vi "Car Main.vi"() -> ()   [LabVIEW 2014]
uses:
  <vilib>/Platform/TimedLoop/XDataNode/timing_clust.ctl
  <vilib>/Platform/TimedLoop/XDataNode/nitl_modes.ctl
  <vilib>/Platform/TimedLoop/XDataNode/wakeup.ctl
  <vilib>/FPGAPlugInAG/sbRIO-9626/niLvFpga_Open_sbRIO-9626.vi
  <vilib>/FPGAPlugInAG/sbRIO-9626/niLvFpga_Reset_sbRIO-9626.vi
  Global Data.vi
  <vilib>/Utility/error.llb/Error Cluster From Error Code.vi
  <vilib>/rvi/errors/niLvFpgaAdjustHostInterfaceError.vi
  <vilib>/FPGAPlugInAG/sbRIO-9626/niLvFpga_Close_sbRIO-9626.vi
  <vilib>/rvi/interface/nirviOpenFPGA/nirviOpenFPGA.xnode
  FPGA Bitfiles/FormulaElectric2_FPGATarget_FPGA_8a5J0mMac2U.lvbitx
  <vilib>/rvi/interface/nirviMethod/nirviMethod.xnode
  <vilib>/Platform/TimedLoop/XDataNode/XDataNode.xnode
  <vilib>/rvi/interface/nirviReadWriteControl/nirviReadWriteControl.xnode
  <vilib>/rvi/interface/nirviCloseFPGA/nirviCloseFPGA.xnode
  <vilib>/NI_Real-Time Target Support.lvlib
  <vilib>/Platform/TimedLoop/XDataNode/XDNodeRunTimeDep.lvlib
  NiFpgaLv.dll
panel:
  in  "baud rate (125000 bps)":u32=250000
  in  "Shutdown":bool
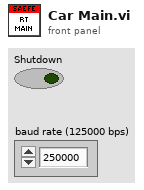
[diagram p1: front panel]
types:
  T1 = typedef "XDNodeRunTimeDep.lvlib/timing_clust.ctl" = cluster{"Expected End [f-1]":u64, "Actual End [f-1]":u64, "Finished Late? [f-1]":bool, "Expected End [i-1]":u64, "Actual End [i-1]":u64, "Finished Late? [i-1]":bool, "Expected Start [i]":u64, "Actual Start [i]":u64, "Expected Start [f]":u64, "Actual Start [f]":u64, "Source Name":string, "Structure Name":string, "Period":i64, "Deadline":i64, "Offset":i64, "Start":i64, "Priority":i32, "Timeout":i32, "Mode":T2, "Wakeup Reason":T3, "Error":errorcluster, "Source Type":string, "Secondary Source Type":string, "Global End Time":u64, "Global Start Time":u64, "Frame Duration":u64, "Iteration Duration":u64, "Assigned CPU":i32, "I/O Scan Engine Mode":u32}
  T2 = typedef "XDNodeRunTimeDep.lvlib/nitl_modes.ctl" = enum32{"No Change", "Process missed periods, maintain original phase", "Discard missed periods, maintain original phase", "Process missed periods, ignore original phase", "Discard missed periods, ignore original phase"}
  T3 = typedef "XDNodeRunTimeDep.lvlib/wakeup.ctl" = enum32{"Normal", "Aborted", "Asynchronous wakeup", "Timing source error", "Timed loop error", "Timeout"}
  T4 = typedef "Remote Stop Type.ctl" = cluster{"bRemoteStop":bool, "bRemoteEmergencyStop":bool, "bRemoteReturnToPits":bool, "bRemoteNewLogs":bool}
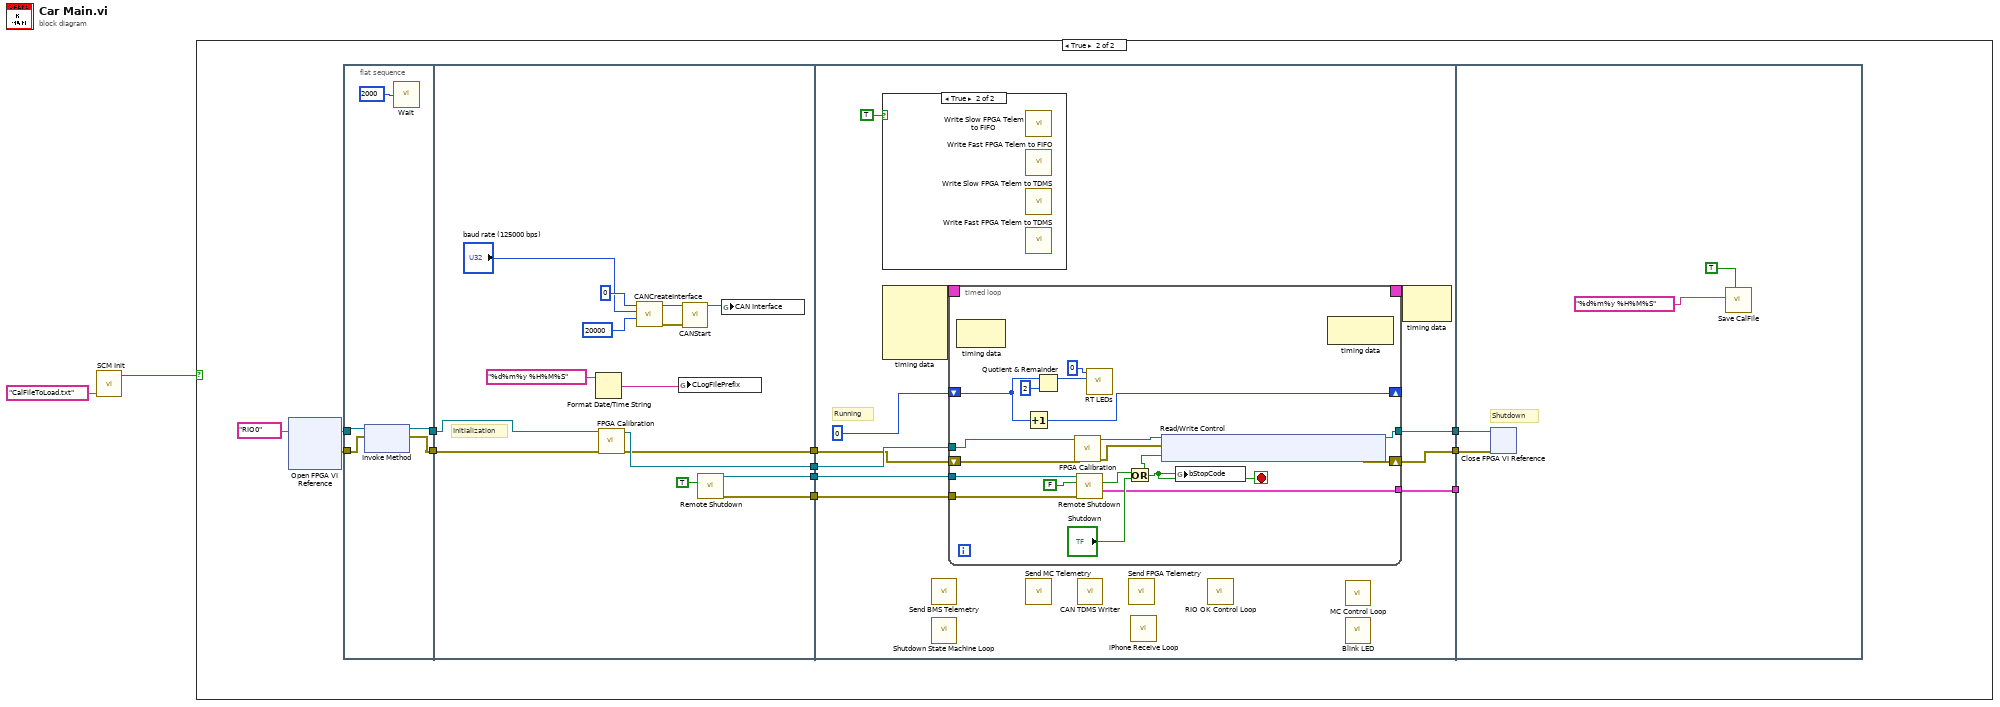
[diagram p0: block diagram]
diagram:
  n1 = call "SCM Init"("Calibration File"="CalFileToLoad.txt") -> ("InitOK"=w2:bool)  [unwired: 2 in, 2 out]
  n2 = case shown="True" w2 {
    frame False {
    }
    frame True {
      n3 = xnode "Open FPGA VI Reference"("resource name"=tag "RIO0") -> ("FPGA VI Reference Out"=w5:refnum<k20>, "error out"=w4:errorcluster)  [unwired: 1 in]
      n4 = flat-sequence {
        tunnel: w4 -> [w17]
        tunnel: w5 -> [w18]
        tunnel: [w16] -> w14
        tunnel: [w15] -> w13
        tunnel: [w21] -> w12
        tunnel: [w20] -> w11
        tunnel: [w33] -> w10
        tunnel: [w32] -> w9
        tunnel: w14 -> [w23]
        tunnel: w13 -> [w22]
        tunnel: w12 -> [w45]
        tunnel: w11 -> [w44]
        tunnel: w10 -> [w42]
        tunnel: w9 -> [w41]
        tunnel: [w40] -> w8
        tunnel: [w37] -> w7
        tunnel: [w36] -> w6
        tunnel: w8 -> [_]
        tunnel: w7 -> [w71]
        tunnel: w6 -> [w70]
        frame #0 {
          n5 = xnode "Invoke Method"("FPGA VI Reference In"=w18, "error in"=w17) -> ("FPGA VI Reference Out"=w16:refnum<k20>, "error out"=w15:errorcluster)
          n6 = call "Wait"("Count(mSec)"=u32 2000) -> ()  [unwired: 1 out]
        }
        frame #1 {
          # "Initialization"
          n7 = Format Date/Time String(time format string (%c)="%d%m%y %H%M%S") -> (date/time string=w24:string)  [unwired: 2 in]
          n8 = call "FPGA Calibration.vi"("error in"=w22, "FPGA VI Reference"=w23) -> ("error out"=w20:errorcluster, "FPGA VI Reference Out"=w21:refnum<k20>)  [unwired: 8 in]
          n9 = call <vilib>:"CANCreateInterface.vi"("receive queue size (5)"=u32 20000, "baud rate (125000 bps)"="baud rate (125000 bps)", "interface index"=u32 0) -> ("error out"=w29:errorcluster, "interface object out"=w28:refnum<k20>)  [unwired: 7 in]
          n10 = global write "Global Data.vi" "CLogFilePrefix"(w24) -> ()
          n11 = call <vilib>:"CANStart.vi"("error in (no error)"=w29, "interface object in"=w28) -> ("interface object out"=w26:refnum<k20>)  [unwired: 8 in, 1 out]
          n12 = call "Remote Shutdown.vi"("Init?"=TRUE) -> ("error out 2"=w32:errorcluster, "port 2"=w33:refnum<k16>)  [unwired: 7 in, 2 out]
          n13 = global write "Global Data.vi" "CAN Interface"(w26) -> ()
        }
        frame #2 {
          # "Running"
          n14 = case shown="True" TRUE {
            frame False {
            }
            frame True {
              n15 = call "Write Slow FPGA Telem to FIFO.vi"() -> ()  [unwired: 12 in]
              n16 = call "Write Fast FPGA Telem to FIFO.vi"() -> ()  [unwired: 12 in]
              n17 = call "Write Slow FPGA Telem to TDMS.vi"() -> ()  [unwired: 12 in]
              n18 = call "Write Fast FPGA Telem to TDMS.vi"() -> ()  [unwired: 12 in]
            }
          }
          n19 = node-c288() -> (w39:T1)  [unwired: 4 in]
          n20 = call "Send BMS Telemetry.vi"() -> ()  [unwired: 12 in]
          n21 = call "Shutdown State Machine Loop.vi"() -> ()  [unwired: 12 in]
          n22 = timed-loop {
            tunnel: w45 -> [w49]
            shift-right: [w59] -> _
            shift-left: 0 ("LED Num") -> [w58]
            tunnel: w42 -> [w55]
            tunnel: w41 -> [w54]
            tunnel: [w52] -> w40
            timing: w39 -> [_]
            timing-out: [_] -> w38
            tunnel: [w51] -> w37
            shift-right: [w50] -> w36
            shift-left: w44 -> [w48]
            stop <- w63 stop-if-true
            n23 = node-c288() -> ()  [unwired: 1 in, 1 out]
            n24 = Increment(x=w58) -> (x+1=w59:i32)
            n25 = Quotient & Remainder(x=w58, y=2) -> (x-y*floor(x/y)=w56:i32)  [unwired: 1 out]
            n26 = call "FPGA Calibration.vi"("error in"=w48, "FPGA VI Reference"=w49) -> ("error out"=w46:errorcluster, "FPGA VI Reference Out"=w47:refnum<k20>)  [unwired: 8 in]
            n27 = call "Remote Shutdown.vi"("error out"=w54, "Init?"=FALSE, "port"=w55) -> ("REMOTE STOP"=w52:T4, "Shutdown?"=w61:bool)  [unwired: 5 in, 2 out]
            n28 = call <vilib>:"RT LEDs.vi"("State"=w56, "LED Num"=0) -> ()  [unwired: 4 in, 2 out]
            n29 = Or(x=w61, y="Shutdown") -> (x .or. y?=w63:bool)
            n30 = xnode "Read/Write Control"("FPGA VI Reference In"=w47, "error in"=w46, "stop"=w63) -> ("FPGA VI Reference Out"=w51:refnum<k20>, "error out"=w50:errorcluster)
            n31 = global write "Global Data.vi" "bStopCode"(w63) -> ()
            n32 = node-c288() -> ()  [unwired: 1 in, 1 out]
          }
          n33 = call "Send MC Telemetry.vi"() -> ()  [unwired: 12 in]
          n34 = call "CAN TDMS Writer.vi"() -> ()  [unwired: 12 in]
          n35 = call "Send FPGA Telemetry.vi"() -> ()  [unwired: 12 in]
          n36 = call "iPhone Receive Loop.vi"() -> ()  [unwired: 12 in]
          n37 = call "RIO OK Control Loop.vi"() -> ()  [unwired: 12 in]
          n38 = call "MC Control Loop.vi"() -> ()  [unwired: 12 in]
          n39 = call "Blink LED.vi"() -> ()  [unwired: 12 in]
          n40 = node-c288(w38) -> ()  [unwired: 1 out]
        }
        frame #3 {
          # "Shutdown"
          n41 = xnode "Close FPGA VI Reference"("FPGA VI Reference In"=w71, "error in"=w70) -> ()  [unwired: 1 out]
          n42 = call <vilib>:"Save CalFile.vi"("Controls Only (F)"=TRUE, "Calibration File"="%d%m%y %H%M%S" ("time format string (%c)")) -> ()  [unwired: 9 in, 1 out]
        }
      }
    }
  }
